vi "Clear Self.vi"(8 "error in (no error)":errorcluster, 10 "Picture in":picture, 11 "Line in":refnum<class "Line.lvclass">) -> (0 "error out":errorcluster, 2 "Picture out":picture, 3 "Line out":refnum<class "Line.lvclass">)   [LabVIEW 2015, in "Line.lvclass"]
uses:
  Line.lvclass
  Graphic/Graphic.lvclass/Graphic.ctl
  Graphic/Graphic.lvclass
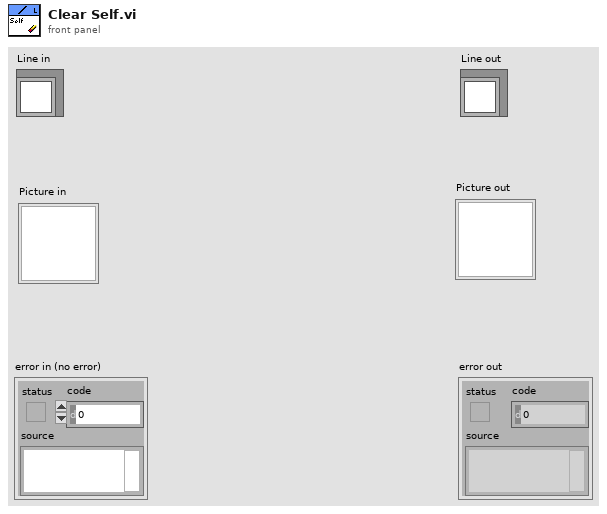
[diagram p1: front panel]
types:
  T1 = cluster{"Width":u16, "Style":enum32{"Solid", "Dash", "Dot", "DashDot", "DashDotDot"}}
  T2 = typedef "Graphic.lvclass/Style.ctl" = cluster{"Color":u32, "Pen":cluster{"Width":u16, "Style":enum32{"Solid", "Dash", "Dot", "DashDot", "DashDotDot"}}}
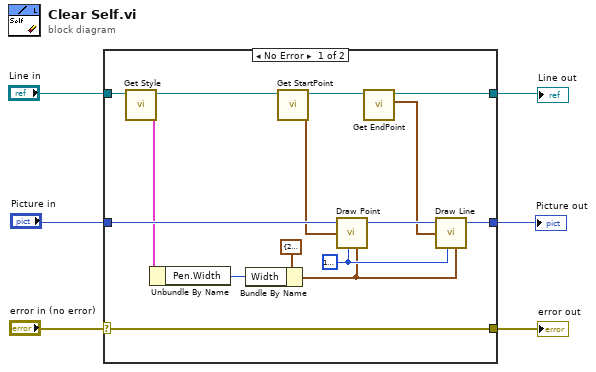
[diagram p0: block diagram]
diagram:
  n1 = case shown="No Error" "error in (no error)" {
    selector: "error in (no error)" -> [w21 w24]
    tunnel: "Line in" -> [w17 w23]
    tunnel: [w15 w23] -> w5
    tunnel: "Picture in" -> [w20 w22]
    tunnel: [w18 w22] -> w3
    tunnel: [w21 w24] -> w2
    frame No Error {
      w12 = u32 16777226 ("Color")
      n2 = call "Get Style.vi"("Graphic in"=w17) -> ("Style"=w10:T2, "Graphic out"=w11:refnum<class "Line.lvclass">)  [unwired: 8 in, 1 out]
      n3 = Unbundle By Name(w10) -> ("Pen.Width"=w8:u16)
      n4 = Bundle By Name(cluster=T1 {"Width"=2, "Style"=enum."Solid"} ("pen"), "Width"=w8) -> (w7:T1)
      n5 = call "Get StartPoint.vi"("Graphic in"=w11) -> ("StartPoint"=w13:cluster{"x":i16, "y":i16}, "Graphic out"=w16:refnum<class "Line.lvclass">)  [unwired: 8 in, 1 out]
      n6 = call <vilib>:"Draw Point.vi"("picture"=w20, "point(x,y)"=w13, "color(black)"=w12, "pen"=w7) -> ("new picture"=w19:picture)  [unwired: 5 in]
      n7 = call "Get EndPoint.vi"("Graphic in"=w16) -> ("EndPoint"=w14:cluster{"x":i16, "y":i16}, "Graphic out"=w15:refnum<class "Line.lvclass">)  [unwired: 8 in, 1 out]
      n8 = call <vilib>:"Draw Line.vi"("picture"=w19, "end point"=w14, "color(black)"=w12, "pen"=w7) -> ("new picture"=w18:picture)  [unwired: 5 in]
    }
    frame Error {
    }
  }
  "error out" <- w2
  "Line out" <- w5
  "Picture out" <- w3
